vi "Query Meas name.vi"(6 "NEXT By Trace":bool, 7 "VISA resource name":refnum<visa-resource-name>="TCPIP0::A-N5224A-41544.local::hislip0::INSTR", 8 "VNA Model":enum16{"E5071C", "N5230A(C)"}(ring)=enum."N5230A(C)", 9 "Channel":string="1") -> (0 "Parameter item":string[](array[string]), 1 "Name list":string[](array[string]), 3 "Dup VISA resource name":refnum<visa-resource-name>)   [LabVIEW 2011]
panel:
  out "Read buffer":string
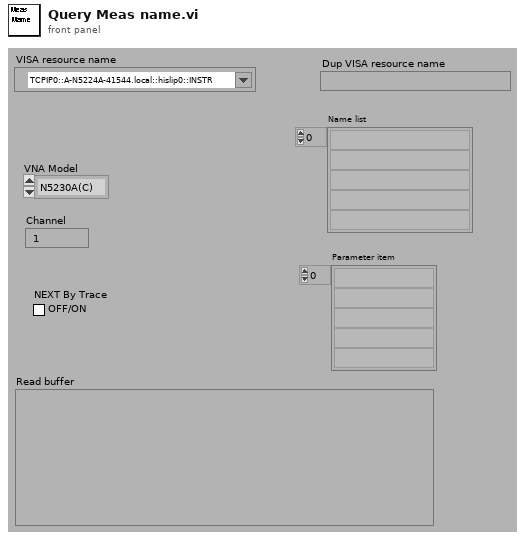
[diagram p1: front panel]
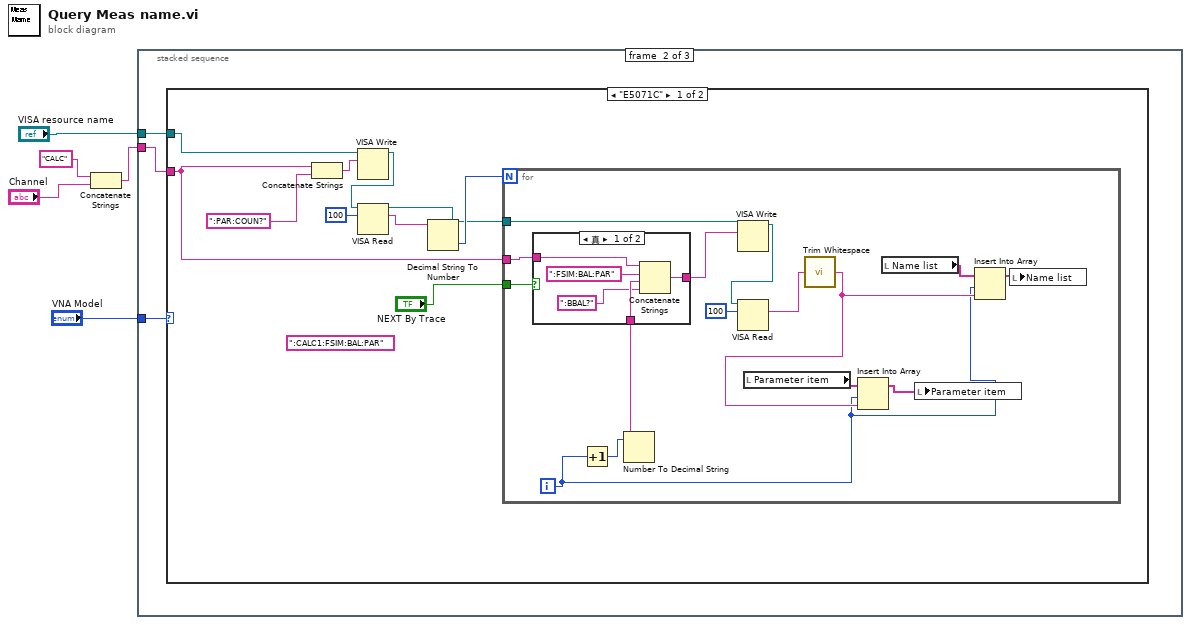
[diagram p0: block diagram]
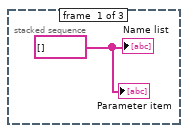
[diagram p2: hidden frame]
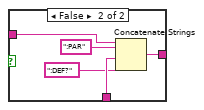
[diagram p3: hidden frame]
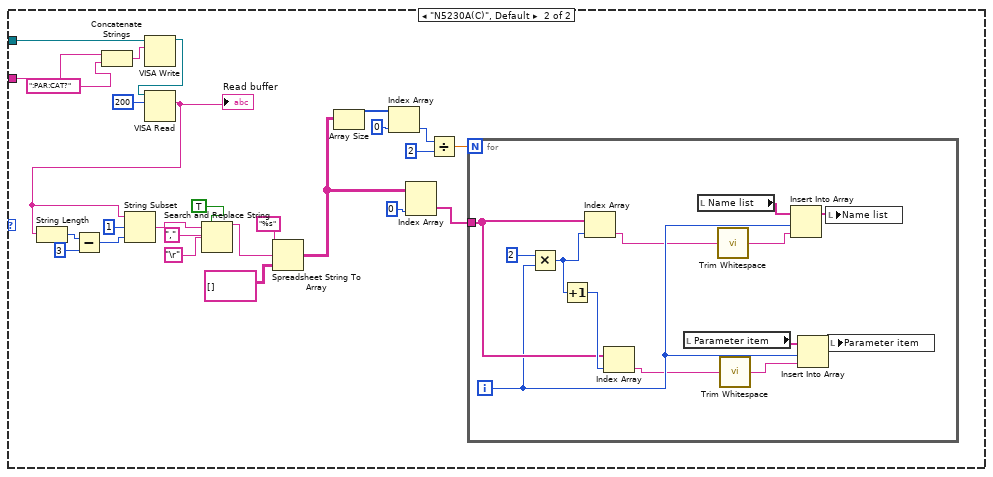
[diagram p4: hidden frame]
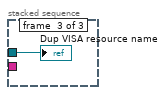
[diagram p5: hidden frame]
diagram:
  n1 = Concatenate Strings("CALC" ("字符串"), "Channel") -> (w2:string)
  n2 = stacked-sequence {
    tunnel: "VISA resource name" -> [_ w9 w84]
    tunnel: "VNA Model" -> [_ w8 _]
    tunnel: w2 -> [_ w7 _]
    frame #0 {
      w6 = string[] [] ("Name list")
      "Name list" <- w6
      "Parameter item" <- w6
    }
    frame #1 {
      n3 = case shown="\"E5071C\"" w8 {
        tunnel: w9 -> [w18 w51]
        tunnel: w7 -> [w11 w45]
        frame "E5071C" {
          (unwired) ":CALC1:FSIM:BAL:PAR" ("string")
          n4 = Concatenate Strings(w11, ":PAR:COUN?") -> (w13:string)
          n5 = VISA Write(VISA resource name=w18, write buffer=w13) -> (VISA resource name out=w17:refnum<visa-resource-name>)  [unwired: 1 in, 2 out]
          n6 = VISA Read(VISA resource name=w17, byte count=u32 100) -> (VISA resource name out=w14:refnum<visa-resource-name>, read buffer=w16:string)  [unwired: 1 in, 2 out]
          n7 = Decimal String To Number(string=w16) -> (number=w15:i32)  [unwired: 2 in, 1 out]
          n8 = for {
            N: w15 -> [_]
            tunnel: w14 -> [w34]
            tunnel: w11 -> [w21]
            tunnel: "NEXT By Trace" -> [w20]
            i -> [w22]
            n9 = Increment(x=w22) -> (x+1=w32:i32)
            n10 = Number To Decimal String(number=w32) -> (decimal integer string=w31:string)  [unwired: 1 in]
            n11 = case shown="真" w20 {
              tunnel: [w39 w44] -> w33
              tunnel: w31 -> [w36 w43]
              tunnel: w21 -> [w38 w40]
              frame True {
                n12 = Concatenate Strings(w38, ":FSIM:BAL:PAR" ("string"), w36, ":BBAL?" ("string")) -> (w39:string)
              }
              frame False {
                n13 = Concatenate Strings(w40, ":PAR" ("string"), w43, ":DEF?" ("string")) -> (w44:string)
              }
            }
            n14 = VISA Write(VISA resource name=w34, write buffer=w33) -> (VISA resource name out=w30:refnum<visa-resource-name>)  [unwired: 1 in, 2 out]
            n15 = VISA Read(VISA resource name=w30, byte count=u32 100) -> (read buffer=w26:string)  [unwired: 1 in, 3 out]
            n16 = local read "Parameter item"() -> (w28:string[])
            n17 = call <vilib>:"Trim Whitespace.vi"("string"=w26) -> ("trimmed string"=w23:string)  [unwired: 1 in]
            n18 = Insert Into Array(array=w28, index=w22, new element=w23) -> (w27:string[])
            n19 = local read "Name list"() -> (w24:string[])
            n20 = local write "Parameter item"(w27) -> ()
            n21 = Insert Into Array(array=w24, index=w22, new element=w23) -> (w25:string[])
            n22 = local write "Name list"(w25) -> ()
          }
        }
        frame "N5230A(C)", Default {
          n23 = Concatenate Strings(w45, ":PAR:CAT?") -> (w47:string)
          n24 = VISA Write(VISA resource name=w51, write buffer=w47) -> (VISA resource name out=w49:refnum<visa-resource-name>)  [unwired: 1 in, 2 out]
          n25 = VISA Read(VISA resource name=w49, byte count=u32 200) -> (read buffer=w48:string)  [unwired: 1 in, 3 out]
          "Read buffer" <- w48
          n26 = String Length(string=w48) -> (length=w63:i32)
          n27 = Subtract(x=w63, y=3) -> (x-y=w61:i32)
          n28 = String Subset(string=w48, offset (0)=1, length (rest)=w61) -> (substring=w60:string)
          n29 = Search and Replace String(replace all?=TRUE ("replace all? (F)"), input string=w60, search string=",", replace string="\r") -> (result string=w68:string)  [unwired: 4 in, 3 out]
          n30 = Spreadsheet String To Array(format string="%s", spreadsheet string=w68, array type (2D Dbl)=string[][] [] ("array 2")) -> (array=w57:string[][])  [unwired: 1 in]
          n31 = Array Size(array=w57) -> (size(s)=w59:i32[])
          n32 = Index Array(array=w59, index=0) -> (element=w54:i32)
          n33 = Index Array(array=w57, index (col)=0 ("disabled index (col)")) -> (element=w55:string[])  [unwired: 1 in]
          n34 = Divide(x=w54, y=2) -> (x/y=w52:dbl)
          n35 = for {
            N: w52 -> [_]
            tunnel: w55 -> [w78]
            i -> [w77]
            n36 = Multiply(x=2, y=w77) -> (x*y=w80:i32)
            n37 = Increment(x=w80) -> (x+1=w79:i32)
            n38 = Index Array(array=w78, index=w80) -> (element=w72:string)
            n39 = Index Array(array=w78, index=w79) -> (element=w74:string)
            n40 = local read "Parameter item"() -> (w76:string[])
            n41 = local read "Name list"() -> (w81:string[])
            n42 = call <vilib>:"Trim Whitespace.vi"("string"=w72) -> ("trimmed string"=w71:string)  [unwired: 1 in]
            n43 = call <vilib>:"Trim Whitespace.vi"("string"=w74) -> ("trimmed string"=w73:string)  [unwired: 1 in]
            n44 = Insert Into Array(array=w81, index=w77, new element=w71) -> (w82:string[])
            n45 = Insert Into Array(array=w76, index=w77, new element=w73) -> (w75:string[])
            n46 = local write "Name list"(w82) -> ()
            n47 = local write "Parameter item"(w75) -> ()
          }
        }
      }
    }
    frame #2 {
      "Dup VISA resource name" <- w84
    }
  }
